vi "Moxom.vi"() -> ()   [LabVIEW 2011]
doc: "This the Rose-Hulman Robotics Tream IGVC compatition Code\nexample demonstrates the control of an autonomous robot through multiple asynchronous processes, modeled by VIs, that communicate with each other using shared variables. This example also shows an obstacle avoidance algorithm that the simulated robot uses as it navigates. The application includes the following processes:\n\n1. LIDAR Loop (\"Sense\")--Uses LabVIEW dataflow programming to generate simulated sensor data based on the position of the robot and any obstacles in the environment.\n\n2. Operator Loop (\"Think\")--Uses a state machine to control the movement of the robot according to commands from the user. When the robot follows a path without joystick or keyboard control, this process controls the attitude of the autonomous robot using a Vector Field Histogram (VFH) algorithm to avoid obstacles.\n\n3. Motor Loop (\"Act\")--Uses a Control and Simulation Loop, from the Control Design and Simulation Module, to create a model of the robot, simulate its dynamic behavior, and show the control loops and attitude observers."
uses:
  <vilib>/robotics/Controls/Compass Indicator/Compass Indicator.xctl
  <vilib>/Platform/TimedLoop/XDataNode/timing_clust.ctl
  <vilib>/Platform/TimedLoop/XDataNode/nitl_modes.ctl
  <vilib>/Platform/TimedLoop/XDataNode/wakeup.ctl
  <vilib>/Platform/TimedLoop/XDataNode/XDataNode.xnode
  <vilib>/Platform/TimedLoop/XDataNode/XDNodeRunTimeDep.lvlib
panel:
  out "Error":bool
  out "OK":bool
  in  "HUD 2":enum32{"GPS", "LIDAR", "IMU", "Occupancy Grid"}(tab)
  out "Health":u8(slide) scale=0.0..12.0
  out "XY Graph 2":cluster{dbl[], dbl[]}(graph)
  out "Data Aquired 2":picture
  out "Digree 2":dbl=16.3201904296875 caption="Digree"
  out "Compass Indicator 2":dbl(xcontrol)=16.3201904296875
  out "Occupancy Grid":dbl[][](graph)
  in  "Telemetry":T1(tab)
  out "Voltage":cluster{sgl, sgl, sgl}(knob)={13.4, 12.0, 47.48} caption="Main Battery Voltage\nInternal Voltage\nDSUB Voltage" scale=8.0..15.0
  out "Current":cluster{sgl, sgl, sgl, sgl}(knob)={0.0, 0.0, -2.0, -2.0} caption="Ch1 Motor Curret\nCh2 Motor Curret\nCh1 Battery Curret \nCh2 Battery Curret" scale=0.0..15.0
  out "IC Temp (C)":i32(slide)=22 scale=0.0..150.0
  out "Ch1 Temp (C)":i32(slide)=22 scale=0.0..150.0
  out "Ch2 Temp (C)":i32(slide)=23 scale=0.0..150.0
  out "Ch1 Encoder Speed\nCh2 Encoder Speed":cluster{i32, i32}(knob) scale=-300.0..300.0
  out "Image Out":T2(plugin-control)
  in  "Search For VISA":bool
  in  "Max RPM/Effort":i32(slide) scale=0.0..1000.0
  in  "HUD":T3(tab)=enum."Info"
  in  "Analog Stick":cluster{dbl, dbl}[](graph)
  in  "Clear Breadcrumbs":bool
  in  "Max Points":dbl=3000.0 format="%0.2f"
  out "XY Graph":cluster{dbl[], dbl[]}[](graph)
  out "Longitude Point":dbl format="%#_12g"
  out "Latitude Point":dbl format="%#_12g"
  out "Data Aquired":picture
  in  "Max Distance":dbl=3000.0 format="%0.2f"
  out "Digree":dbl=16.3201904296875
  out "Compass Indicator":dbl(xcontrol)=16.3201904296875
  out "Curretn POI":string
  in  "Curent Index":i32
  in  "Waypoint Table":string[][](table)=[["1.000000", "39.400000", "-87.200000"], ["2.000000", "39.600000", "-87.300000"], ["2.000000", "39.200000", "-87.400000"]]
  in  "Show GPS Diagram":bool
  in  "Show LL Diagram":bool
  in  "Show OL Diagram":bool
  in  "Show MCL Diagram":bool
  in  "VFH Visualization":bool
  in  "About":bool
  in  "Stop":bool
  in  "Error Display":T4(tab)
  out "Cammera Status":bool
  out "Cammera Status 2":bool
  out "IMU Status":bool
  in  "IMU VISA":refnum<visa-resource-name>="COM7"
  out "Motor Status":bool
  in  "Motor VISA":refnum<visa-resource-name>="COM21"
  out "LIDAR Status":bool
  in  "LIDAR VISA":refnum<visa-resource-name>="COM20"
  out "GPS Status":bool
  in  "GPS VISA":refnum<visa-resource-name>="COM22"
  in  "GPS Error":errorcluster
  in  "LIDAR Error":errorcluster
  in  "Motor Error":errorcluster
  in  "IMU Error":errorcluster
  in  "Camera Error":errorcluster
  in  "Robot Mode:":T5(ring)
  out "End Loop":bool=TRUE
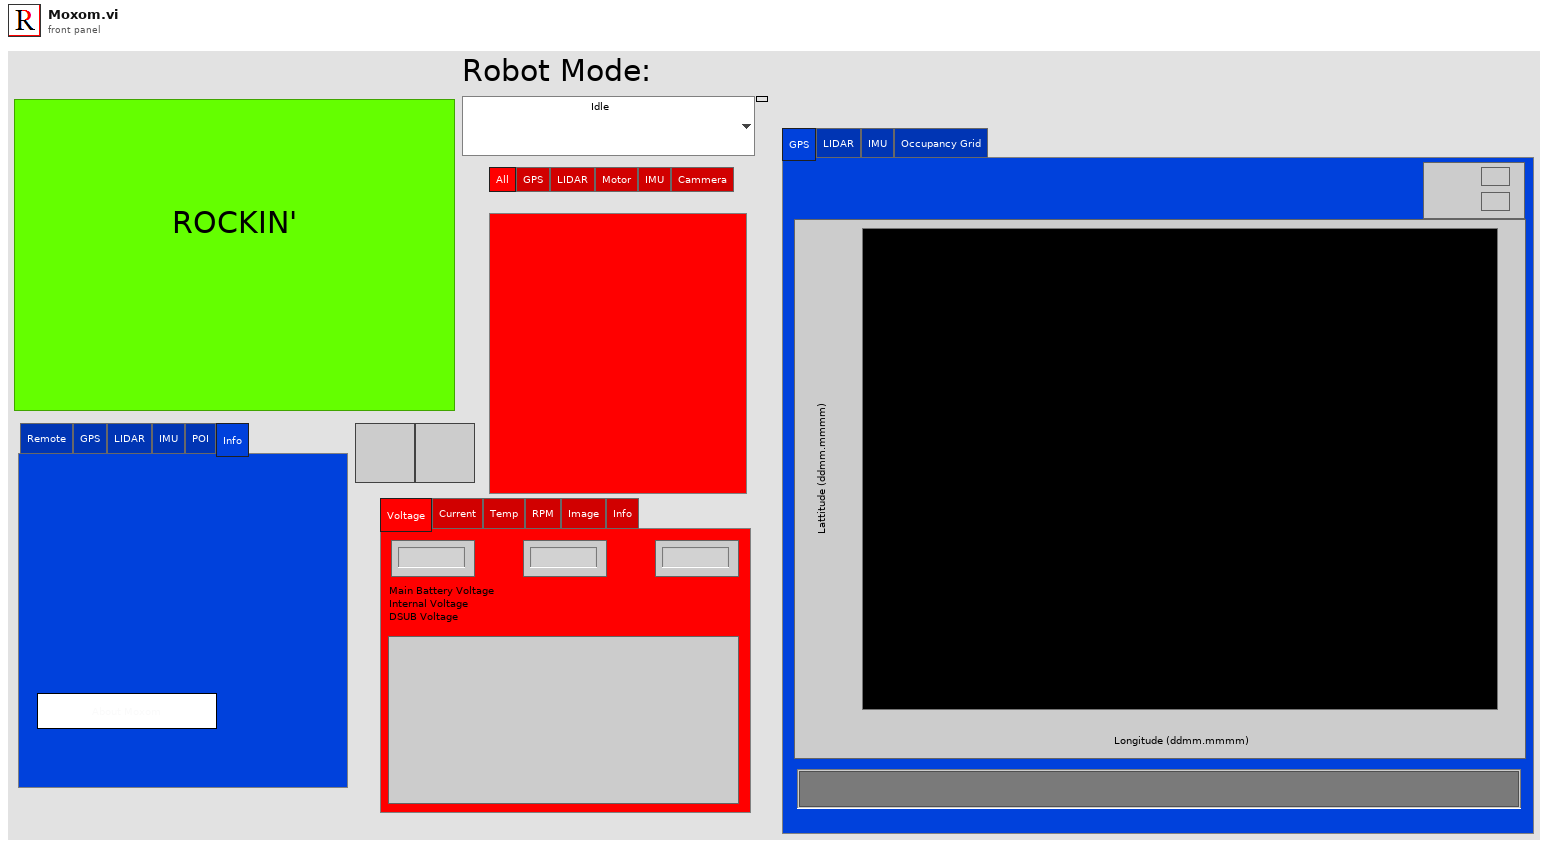
[diagram p1: front panel]
types:
  T1 = enum32{"Voltage", "Current", "Temp", "RPM", "Image", "Info"}
  T2 = typedef "IMAQ Image.ctl" = refnum<image>
  T3 = enum32{"Remote", "GPS", "LIDAR", "IMU", "POI", "Info"}
  T4 = enum32{"All", "GPS", "LIDAR", "Motor", "IMU", "Cammera"}
  T5 = enum16{"Idle", "Wiimote", "Joypad", "IGVC", "Avoide Objects", "Avoide Lines", "Path Planning", "Heading", "Waypoint"}
  T6 = cluster{"Latitude":dbl, "Longitude":dbl, "Altitude":dbl, "Velocity, Correction & SET":cluster{"Velocity North":dbl, "Velocity East":dbl, "Velocity Up":dbl, "Ellipsoidal Height":dbl, "GDOP":sgl, "PDOP":sgl, "HDOP":sgl, "VDOP":sgl, "TDOP":sgl, "Horizontal Figure of Merit":u8, "Time Figure of Merit":u8, "Max dGPS Age":sgl, "Extended Navigation Mode":u8, "Antenna Height Adjustment ":dbl, "SET North":i32, "SET East":i32, "SET Up":i32}, "Time":cluster{"GPS Week":u16, "GPS Time of Week":sgl}, "Satellites Used":i32[]}
  T7 = typedef "XDNodeRunTimeDep.lvlib/timing_clust.ctl" = cluster{"Expected End [f-1]":u64, "Actual End [f-1]":u64, "Finished Late? [f-1]":bool, "Expected End [i-1]":u64, "Actual End [i-1]":u64, "Finished Late? [i-1]":bool, "Expected Start [i]":u64, "Actual Start [i]":u64, "Expected Start [f]":u64, "Actual Start [f]":u64, "Source Name":string, "Structure Name":string, "Period":i64, "Deadline":i64, "Offset":i64, "Start":i64, "Priority":i32, "Timeout":i32, "Mode":T8, "Wakeup Reason":T9, "Error":errorcluster, "Source Type":string, "Secondary Source Type":string, "Global End Time":u64, "Global Start Time":u64, "Frame Duration":u64, "Iteration Duration":u64, "Assigned CPU":i32, "I/O Scan Engine Mode":u32}
  T8 = typedef "XDNodeRunTimeDep.lvlib/nitl_modes.ctl" = enum32{"No Change", "Process missed periods, maintain original phase", "Discard missed periods, maintain original phase", "Process missed periods, ignore original phase", "Discard missed periods, ignore original phase"}
  T9 = typedef "XDNodeRunTimeDep.lvlib/wakeup.ctl" = enum32{"Normal", "Aborted", "Asynchronous wakeup", "Timing source error", "Timed loop error", "Timeout"}
  T10 = cluster{"Position":cluster{"Roll":dbl, "Pitch":dbl, "Yaw":dbl}, "Orientation Matrix":dbl[][], "Magnetic Field":cluster{"Z-Axis Magnetic Field":dbl, "Y-Axis Magnetic Field":dbl, "X-Axis Magnetic Field":dbl}, "Acceleration":cluster{"Z-Axis Acceleration":dbl, "Y-Axis Acceleration":dbl, "X-Axis Acceleration":dbl}, "Angular Rate":cluster{"X-Axis Angular Rate":dbl, "Y-Axis Angular Rate":dbl, "Z-Axis Angular Rate":dbl}, "Quaternion":dbl[]}
  T11 = cluster{"Azimuth":dbl, "FocusPointAltitude":dbl, "altMode":i32, "FocusPointLatitude":dbl, "FocusPointLongitude":dbl, "Range":dbl, "Tilt":dbl}
  T12 = cluster{"Voltage":cluster{sgl, sgl, sgl}, "Encoder Speed":cluster{i32, i32}, "Temps":cluster{"IC Temp (C)":i32, "Ch1 Temp (C)":i32, "Ch2 Temp (C)":i32}, "Current":cluster{dbl, dbl, dbl, dbl}}
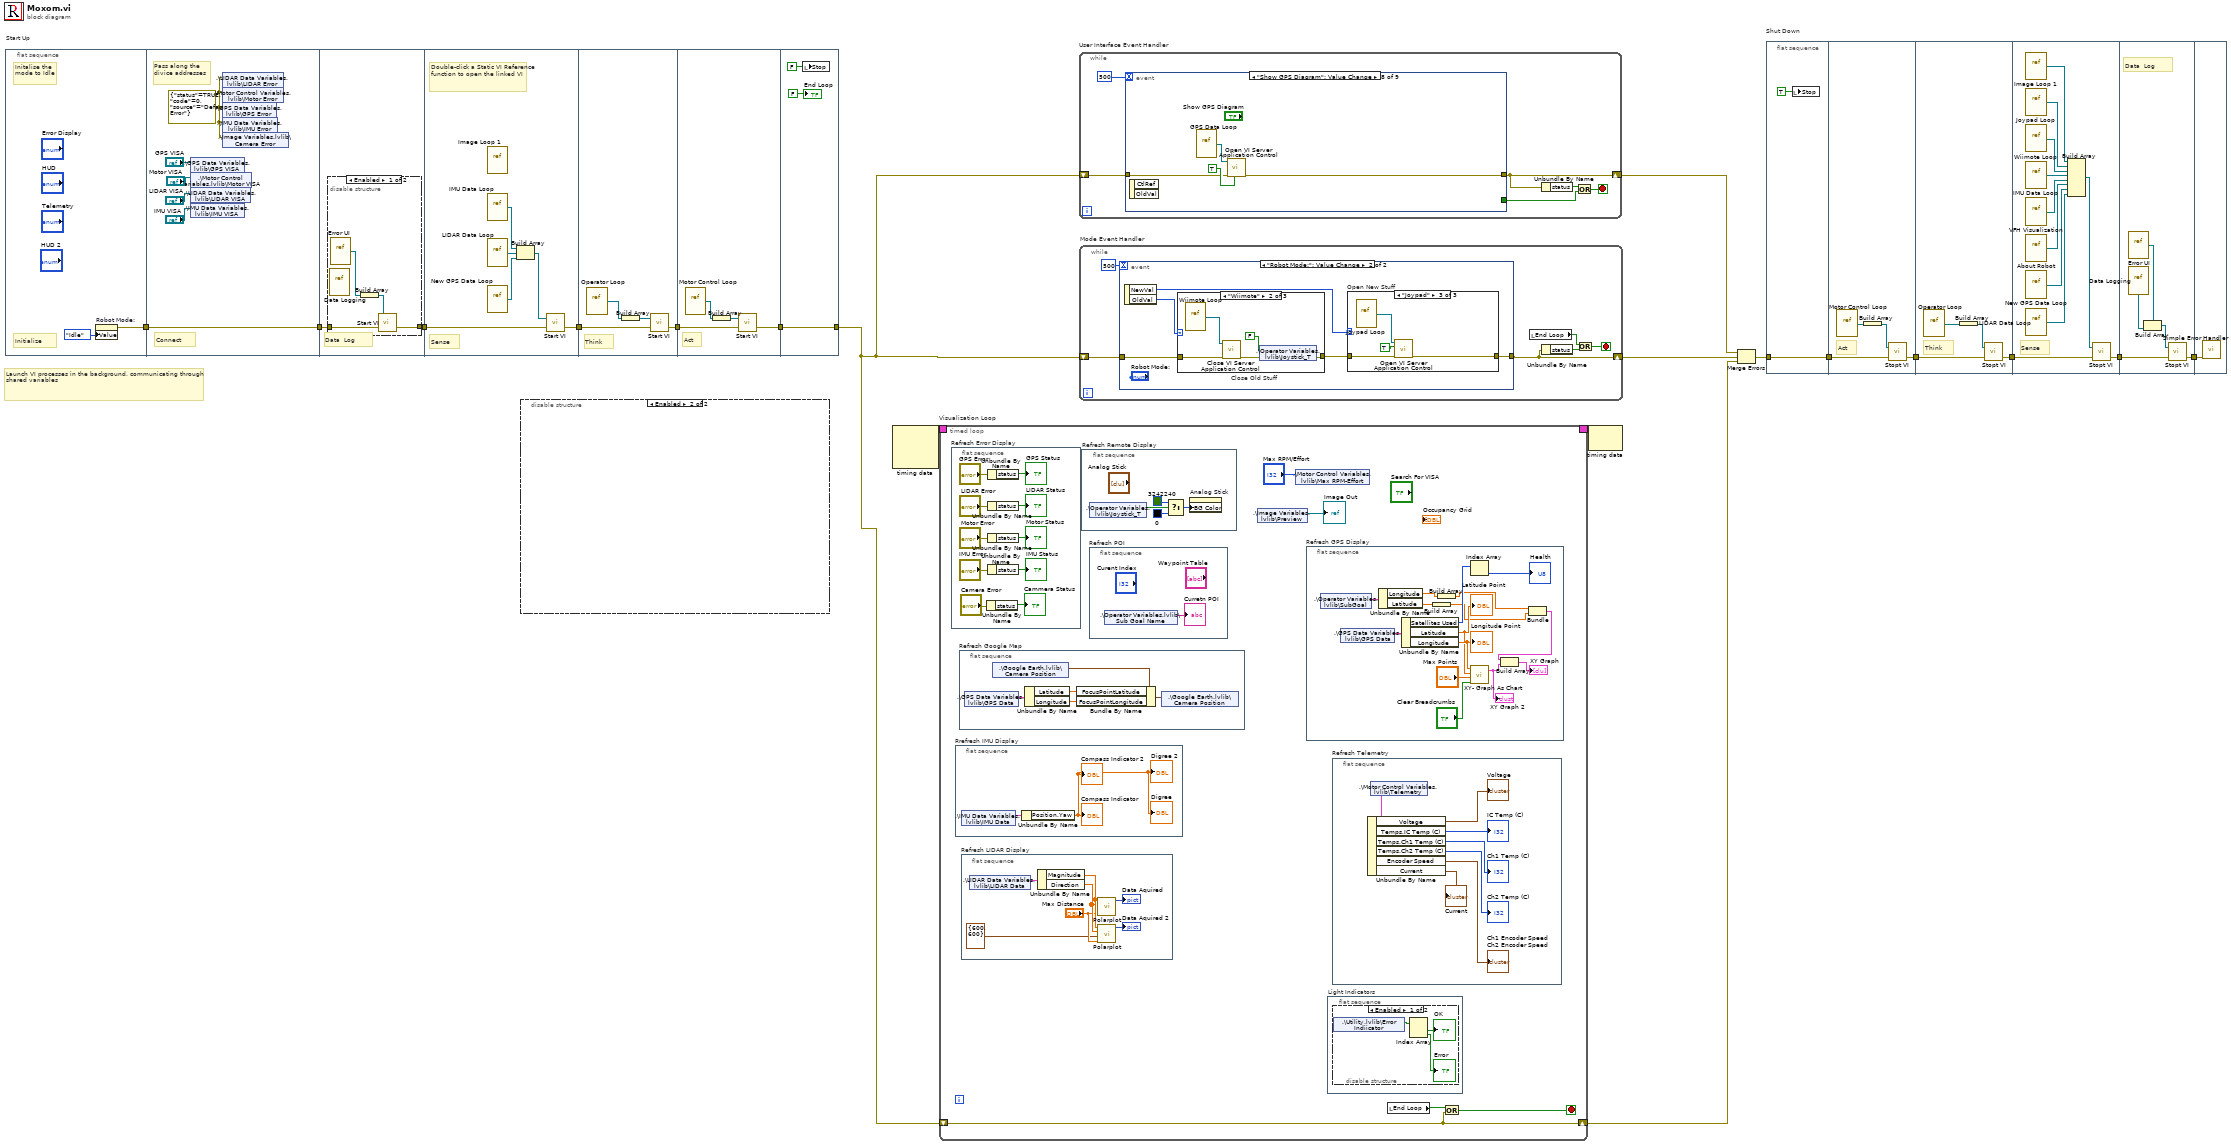
[diagram p0: block diagram]
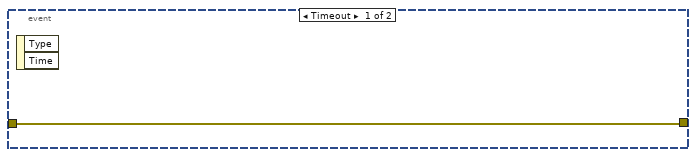
[diagram p2: hidden frame]
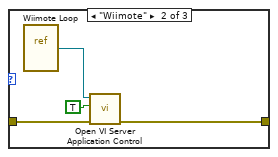
[diagram p4: hidden frame]
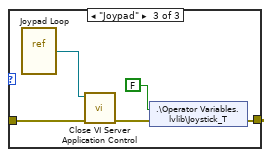
[diagram p6: hidden frame]
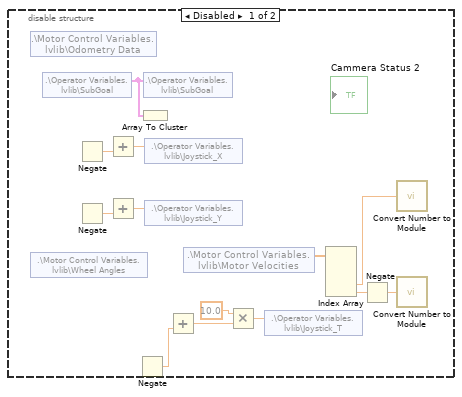
[diagram p7: hidden frame]
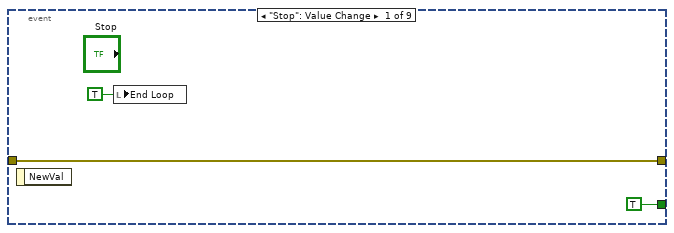
[diagram p9: hidden frame]
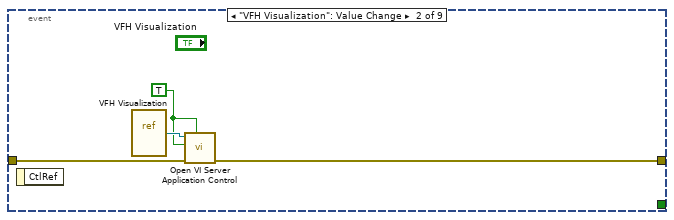
[diagram p10: hidden frame]
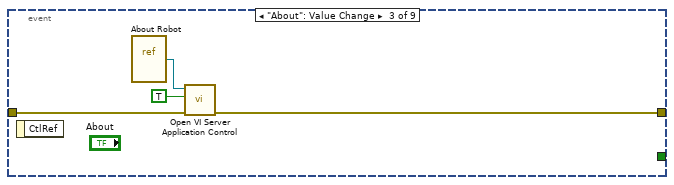
[diagram p11: hidden frame]
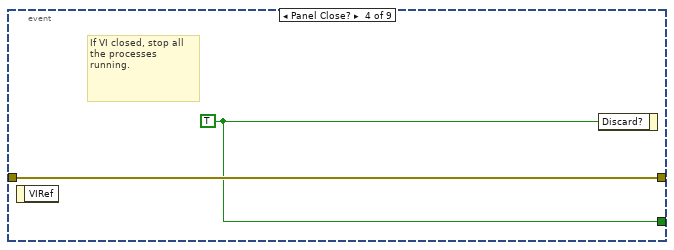
[diagram p12: hidden frame]
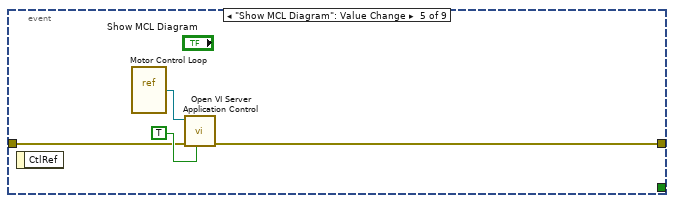
[diagram p13: hidden frame]
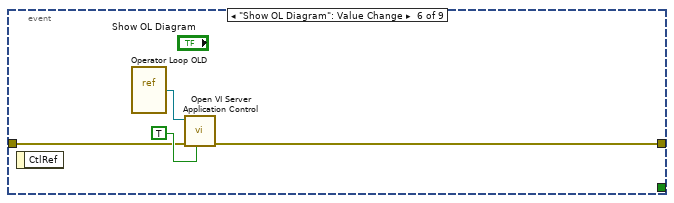
[diagram p14: hidden frame]
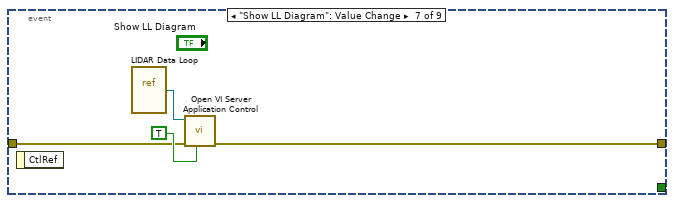
[diagram p15: hidden frame]
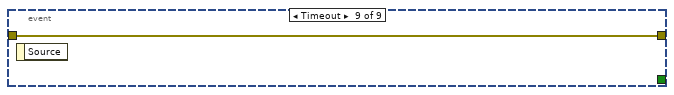
[diagram p16: hidden frame]
diagram:
  # "Launch VI processes in the background, communicating through shared variables"
  n1 = flat-sequence "Start Up" {
    tunnel: [w20] -> w13
    tunnel: [w23] -> w5
    tunnel: w13 -> [w23]
    tunnel: w5 -> [w28]
    tunnel: [w27] -> w1
    tunnel: [w37] -> w12
    tunnel: w1 -> [w38]
    tunnel: w12 -> [w43]
    tunnel: [w42] -> w10
    tunnel: [w46] -> w11
    tunnel: w10 -> [w47]
    tunnel: [w50] -> w6
    tunnel: w11 -> [w50]
    frame #0 {
      # "Initialize"
      # "Initalise the mode to Idle"
      n2 = property on="Robot Mode:" class="Enum (strict)"("Value"=T5."Idle" ("Robot Mode:")) -> (error out=w20:errorcluster)  [unwired: 2 in, 1 out]
    }
    frame #1 {
      w21 = errorcluster {"status"=TRUE, "code"=0, "source"="Default Error"} ("error out")
      # "Connect"
      # "Pass along the divice addresses"
      n3 = shared-variable ".\\GPS Data Variables.lvlib\\GPS VISA"("GPS VISA") -> ()  [unwired: 1 in, 1 out]
      n4 = shared-variable ".\\LIDAR Data Variables.lvlib\\LIDAR VISA"("LIDAR VISA") -> ()  [unwired: 1 in, 1 out]
      n5 = shared-variable ".\\IMU Data Variables.lvlib\\IMU VISA"("IMU VISA") -> ()  [unwired: 1 in, 1 out]
      n6 = shared-variable ".\\Motor Control Variables.lvlib\\Motor VISA"("Motor VISA") -> ()  [unwired: 1 in, 1 out]
      n7 = shared-variable ".\\LIDAR Data Variables.lvlib\\LIDAR Error"(w21) -> ()  [unwired: 1 in, 1 out]
      n8 = shared-variable ".\\Motor Control Variables.lvlib\\Motor Error"(w21) -> ()  [unwired: 1 in, 1 out]
      n9 = shared-variable ".\\GPS Data Variables.lvlib\\GPS Error"(w21) -> ()  [unwired: 1 in, 1 out]
      n10 = shared-variable ".\\IMU Data Variables.lvlib\\IMU Error"(w21) -> ()  [unwired: 1 in, 1 out]
      n11 = shared-variable ".\\Image Variables.lvlib\\Camera Error"(w21) -> ()  [unwired: 1 in, 1 out]
    }
    frame #2 {
      # "Data  Log"
      n12 = disable-structure shown="Enabled" {
        disable-tunnel: w28 -> [w31 w33]
        disable-tunnel: [w30 w33] -> w27
        frame Enabled {
          n13 = vi-ref "Data Logging.vi"() -> ()  [unwired: 1 out]
          n14 = vi-ref "Error UI.vi"() -> (w29:refnum<vi>)
          n15 = Build Array(w29) -> (w32:refnum<vi>[])
          n16 = call "Start VI.vi"("error in"=w31, "VI refnum"=w32) -> ("error out"=w30:errorcluster)  [unwired: 1 in]
        }
        frame Disabled {
        }
      }
    }
    frame #3 {
      # "Double-click a Static VI Reference function to open the linked VI"
      # "Sense"
      n17 = vi-ref "Image Loop 1.vi"() -> ()  [unwired: 1 out]
      n18 = vi-ref "IMU Data Loop.vi"() -> (w35:refnum<vi>)
      n19 = vi-ref "LIDAR Data Loop.vi"() -> (w36:refnum<vi>)
      n20 = vi-ref "New GPS Data Loop.vi"() -> (w34:refnum<vi>)
      n21 = Build Array(w35, w36, w34) -> (w39:refnum<vi>[])
      n22 = call "Start VI.vi"("error in"=w38, "VI refnum"=w39) -> ("error out"=w37:errorcluster)  [unwired: 1 in]
    }
    frame #4 {
      # "Think"
      n23 = vi-ref "Operator Loop.vi"() -> (w41:refnum<vi>)
      n24 = Build Array(w41) -> (w40:refnum<vi>[])
      n25 = call "Start VI.vi"("error in"=w43, "VI refnum"=w40) -> ("error out"=w42:errorcluster)  [unwired: 1 in]
    }
    frame #5 {
      # "Act"
      n26 = vi-ref "Motor Control Loop.vi"() -> (w45:refnum<vi>)
      n27 = Build Array(w45) -> (w44:refnum<vi>[])
      n28 = call "Start VI.vi"("error in"=w47, "VI refnum"=w44) -> ("error out"=w46:errorcluster)  [unwired: 1 in]
    }
    frame #6 {
      n29 = local write "Stop"(FALSE ("Halt TL")) -> ()
      "End Loop" <- FALSE ("Halt TL")
    }
  }
  n30 = disable-structure shown="Enabled" {
    frame Disabled {
      n31 = shared-variable ".\\Motor Control Variables.lvlib\\Odometry Data"() -> ()  [unwired: 1 in, 2 out]
      n32 = shared-variable ".\\Motor Control Variables.lvlib\\Wheel Angles"() -> ()  [unwired: 1 in, 2 out]
      n33 = shared-variable ".\\Operator Variables.lvlib\\SubGoal"() -> (w51:T6)  [unwired: 1 in, 1 out]
      n34 = Negate() -> (-x=w55:dbl)  [unwired: 1 in]
      n35 = Negate() -> (-x=w56:dbl)  [unwired: 1 in]
      n36 = Add(y=w55) -> (x+y=w65:dbl)  [unwired: 1 in]
      n37 = Add(y=w56) -> (x+y=w64:dbl)  [unwired: 1 in]
      n38 = Negate() -> (-x=w54:dbl)  [unwired: 1 in]
      n39 = Array To Cluster(array=w51) -> ()  [unwired: 1 out]
      n40 = shared-variable ".\\Operator Variables.lvlib\\SubGoal"(w51) -> ()  [unwired: 1 in, 1 out]
      n41 = shared-variable ".\\Operator Variables.lvlib\\Joystick_X"(w65) -> ()  [unwired: 1 in, 1 out]
      n42 = shared-variable ".\\Operator Variables.lvlib\\Joystick_Y"(w64) -> ()  [unwired: 1 in, 1 out]
      n43 = Add(y=w54) -> (x+y=w53:dbl)  [unwired: 1 in]
      n44 = shared-variable ".\\Motor Control Variables.lvlib\\Motor Velocities"() -> (w62:dbl[])  [unwired: 1 in, 1 out]
      n45 = Multiply(x=10.0, y=w53) -> (x*y=w63:dbl)
      n46 = shared-variable ".\\Operator Variables.lvlib\\Joystick_T"(w63) -> ()  [unwired: 1 in, 1 out]
      n47 = Index Array(array=w62) -> (element #3=w59:dbl, element #4=w58:dbl)  [unwired: 4 in, 2 out]
      n48 = Negate(x=w58) -> (-x=w57:dbl)
      n49 = call "Convert Number to Module.vi"("input"=w59) -> ("Positive Module"=w60:dbl)  [unwired: 6 in, 1 out]
      n50 = call "Convert Number to Module.vi"("input"=w57) -> ("Positive Module"=w61:dbl)  [unwired: 6 in, 1 out]
    }
    frame Enabled {
    }
  }
  n51 = node-c288() -> (w18:T7)  [unwired: 3 in]
  n52 = timed-loop "Visualization Loop" {
    timing: w18 -> [_]
    timing-out: [_] -> w17
    shift-right: [w66] -> w2
    shift-left: w6 -> [w66]
    stop <- w70 stop-if-true
    n53 = flat-sequence "Refresh Error Display" {
      frame #0 {
        n54 = Unbundle By Name("Camera Error") -> ("status"=→"Cammera Status":bool)
        n55 = Unbundle By Name("GPS Error") -> ("status"=→"GPS Status":bool)
        n56 = Unbundle By Name("LIDAR Error") -> ("status"=→"LIDAR Status":bool)
        n57 = Unbundle By Name("Motor Error") -> ("status"=→"Motor Status":bool)
        n58 = Unbundle By Name("IMU Error") -> ("status"=→"IMU Status":bool)
      }
    }
    n59 = flat-sequence "Rrefresh IMU Display" {
      frame #0 {
        n60 = shared-variable ".\\IMU Data Variables.lvlib\\IMU Data"() -> (w98:T10)  [unwired: 1 in, 1 out]
        n61 = Unbundle By Name(w98) -> ("Position.Yaw"=→"Compass Indicator" →"Digree" →"Compass Indicator 2" →"Digree 2":dbl)
      }
    }
    n62 = flat-sequence "Refresh Google Map" {
      frame #0 {
        n63 = shared-variable ".\\GPS Data Variables.lvlib\\GPS Data"() -> (w109:T6)  [unwired: 1 in, 1 out]
        n64 = shared-variable ".\\Google Earth.lvlib\\Camera Position"() -> (w110:T11)  [unwired: 1 in, 1 out]
        n65 = Unbundle By Name(w109) -> ("Latitude"=w106:dbl, "Longitude"=w108:dbl)
        n66 = Bundle By Name(cluster=w110, "FocusPointLatitude"=w106, "FocusPointLongitude"=w108) -> (w107:T11)
        n67 = shared-variable ".\\Google Earth.lvlib\\Camera Position"(w107) -> ()  [unwired: 1 in, 1 out]
      }
    }
    n68 = flat-sequence "Refresh LIDAR Display" {
      frame #0 {
        n69 = shared-variable ".\\LIDAR Data Variables.lvlib\\LIDAR Data"() -> (w80:cluster{"Magnitude":dbl[], "Direction":dbl[]})  [unwired: 1 in, 1 out]
        n70 = Unbundle By Name(w80) -> ("Magnitude"=w77:dbl[], "Direction"=w76:dbl[])
        n71 = call "Polarplot.vi"("maximum"="Max Distance", "Direction"=w76, "Magnitude"=w77) -> ("Data Aquired"=→"Data Aquired":picture)  [unwired: 8 in]
        n72 = call "Polarplot.vi"("maximum"="Max Distance", "dimensions (w,h)"=cluster{"width":i16, "height":i16} {"width"=600, "height"=600}, "Direction"=w76, "Magnitude"=w77) -> ("Data Aquired"=→"Data Aquired 2":picture)  [unwired: 7 in]
      }
    }
    n73 = flat-sequence "Refresh Remote Display" {
      frame #0 {
        n74 = shared-variable ".\\Operator Variables.lvlib\\Joystick_T"() -> (w112:bool)  [unwired: 1 in, 1 out]
        n75 = Select(t=u32 3242240, s=w112, f=u32 0) -> (s? t:f=w111:u32)
        n76 = property on="Analog Stick" class="XYGraph (strict)"("BG Color"=w111) -> ()  [unwired: 2 in, 2 out]
      }
    }
    n77 = flat-sequence "Refresh POI" {
      frame #0 {
        n78 = shared-variable ".\\Operator Variables.lvlib\\Sub Goal Name"() -> (→"Curretn POI":string)  [unwired: 1 in, 1 out]
      }
    }
    n79 = shared-variable ".\\Image Variables.lvlib\\Preview"() -> (→"Image Out":refnum<image>)  [unwired: 1 in, 1 out]
    n80 = shared-variable ".\\Motor Control Variables.lvlib\\Max RPM-Effort"("Max RPM/Effort") -> ()  [unwired: 1 in, 1 out]
    n81 = flat-sequence "Refresh GPS Display" {
      frame #0 {
        n82 = shared-variable ".\\Operator Variables.lvlib\\SubGoal"() -> (w91:T6)  [unwired: 1 in, 1 out]
        n83 = shared-variable ".\\GPS Data Variables.lvlib\\GPS Data"() -> (w95:T6)  [unwired: 1 in, 1 out]
        n84 = Unbundle By Name(w91) -> ("Longitude"=w86:dbl, "Latitude"=w85:dbl)
        n85 = Unbundle By Name(w95) -> ("Satellites Used"=w92:i32[], "Latitude"=w89:dbl, "Longitude"=w90:dbl)
        "Latitude Point" <- w89
        "Longitude Point" <- w90
        n86 = Build Array(w85) -> (w83:dbl[])
        n87 = Build Array(w86) -> (w84:dbl[])
        n88 = Index Array(array=w92) -> (element=→"Health":i32)  [unwired: 1 in]
        n89 = call "XY- Graph As Chart.vi"("Clear Graph (F)"="Clear Breadcrumbs", "Maxi Points (10,000)"="Max Points", "Y-Value"=w89, "X- Value"=w90) -> ("XY Graph"=w88:cluster{dbl[], dbl[]})  [unwired: 1 out]
        "XY Graph 2" <- w88
        n90 = Bundle(w84, w83) -> (w82:cluster{dbl[], dbl[]})  [unwired: 1 out]
        n91 = Build Array(w82, w88) -> (→"XY Graph":cluster{dbl[], dbl[]}[])
      }
    }
    n92 = flat-sequence "Light Indicators" {
      frame #0 {
        n93 = disable-structure shown="Enabled" {
          frame Enabled {
            n94 = shared-variable ".\\Utility.lvlib\\Error Indiicator"() -> (w73:bool[])  [unwired: 1 in, 1 out]
            n95 = Index Array(array=w73) -> (element #1=→"OK":bool, element #2=→"Error":bool)  [unwired: 2 in]
          }
          frame Disabled {
          }
        }
      }
    }
    n96 = flat-sequence "Refresh Telemetry" {
      frame #0 {
        n97 = shared-variable ".\\Motor Control Variables.lvlib\\Telemetry"() -> (w105:T12)  [unwired: 1 in, 1 out]
        n98 = Unbundle By Name(w105) -> ("Voltage"=→"Voltage":cluster{sgl, sgl, sgl}, "Temps.IC Temp (C)"=→"IC Temp (C)":i32, "Temps.Ch1 Temp (C)"=→"Ch1 Temp (C)":i32, "Temps.Ch2 Temp (C)"=→"Ch2 Temp (C)":i32, "Encoder Speed"=→"Ch1 Encoder Speed\nCh2 Encoder Speed":cluster{i32, i32}, "Current"=→"Current":cluster{dbl, dbl, dbl, dbl})
      }
    }
    n99 = local read "End Loop"() -> (w67:bool)
    n100 = Or(x=w67, y=w66) -> (x .or. y?=w70:bool)
  }
  n101 = while "User Interface Event Handler" {
    shift-right: [w129] -> w16
    shift-left: w6 -> [w132]
    stop <- w131 stop-if-true
    n102 = event shown="[7] \"Show GPS Diagram\": Value Change" {
      selector: _ -> [_ _ _ _ _ _ _ _ _]
      dyn-events: _ -> [_ _ _ _ _ _ _ _ _]
      timeout: 500 -> [_ _ _ _ _ _ _ _ _]
      tunnel: [TRUE _ _ w144 _ _ _ _ _] -> w127
      tunnel: w132 -> [w135 w137 w142 w145 w147 w151 w155 w158 w162]
      tunnel: [w135 w136 w141 w145 w146 w150 w154 w159 w162] -> w129
      event "Stop": Value Change {
        n103 = event-data() -> ()  [unwired: 2 out]
        n104 = local write "End Loop"(TRUE ("End Loop")) -> ()
      }
      event "VFH Visualization": Value Change {
        w138 = TRUE ("Launch Map")
        n105 = event-data() -> ()  [unwired: 2 out]
        n106 = vi-ref "VFH Visualization.vi"() -> (w139:refnum<vi>)
        n107 = call "Open VI Server Application Control.vi"("open front panel (F)"=w138, "error in (no error)"=w137, "run VI (F)"=w138, "VI refnum"=w139) -> ("error out"=w136:errorcluster)  [unwired: 7 in]
      }
      event "About": Value Change {
        n108 = event-data() -> ()  [unwired: 2 out]
        n109 = vi-ref "About Robot.vi"() -> (w143:refnum<vi>)
        n110 = call "Open VI Server Application Control.vi"("error in (no error)"=w142, "run VI (F)"=TRUE ("Launch Map"), "VI refnum"=w143) -> ("error out"=w141:errorcluster)  [unwired: 8 in]
      }
      event Panel Close? {
        w144 = TRUE ("Discard?")
        # "If VI closed, stop all the processes running."
        n111 = event-data() -> ()  [unwired: 2 out]
        n112 = event-data("Discard?"=w144) -> ()  [unwired: 1 in, 1 out]
      }
      event "Show MCL Diagram": Value Change {
        n113 = event-data() -> ()  [unwired: 2 out]
        n114 = vi-ref "Motor Control Loop.vi"() -> (w149:refnum<vi>)
        n115 = call "Open VI Server Application Control.vi"("open block diagram (F)"=TRUE ("Open Front Panel"), "error in (no error)"=w147, "VI refnum"=w149) -> ("error out"=w146:errorcluster)  [unwired: 8 in]
      }
      event "Show OL Diagram": Value Change {
        n116 = event-data() -> ()  [unwired: 2 out]
        n117 = vi-ref "Operator Loop OLD.vi"() -> (w152:refnum<vi>)
        n118 = call "Open VI Server Application Control.vi"("open block diagram (F)"=TRUE ("Open Front Panel"), "error in (no error)"=w151, "VI refnum"=w152) -> ("error out"=w150:errorcluster)  [unwired: 8 in]
      }
      event "Show LL Diagram": Value Change {
        n119 = event-data() -> ()  [unwired: 2 out]
        n120 = vi-ref "LIDAR Data Loop.vi"() -> (w156:refnum<vi>)
        n121 = call "Open VI Server Application Control.vi"("open block diagram (F)"=TRUE ("Open Front Panel"), "error in (no error)"=w155, "VI refnum"=w156) -> ("error out"=w154:errorcluster)  [unwired: 8 in]
      }
      event "Show GPS Diagram": Value Change {
        n122 = event-data() -> ()  [unwired: 3 out]
        n123 = vi-ref "GPS Data Loop.vi"() -> (w160:refnum<vi>)
        n124 = call "Open VI Server Application Control.vi"("open block diagram (F)"=TRUE ("Open Front Panel"), "error in (no error)"=w158, "VI refnum"=w160) -> ("error out"=w159:errorcluster)  [unwired: 8 in]
      }
      event Timeout {
        n125 = event-data() -> ()  [unwired: 2 out]
      }
    }
    n126 = Unbundle By Name(w129) -> ("status"=w128:bool)
    n127 = Or(x=w128, y=w127) -> (x .or. y?=w131:bool)
  }
  n128 = while "Mode Event Handler" {
    shift-right: [w165] -> w7
    shift-left: w6 -> [w166]
    stop <- w167 stop-if-true
    n129 = event shown="[1] \"Robot Mode:\": Value Change" {
      selector: _ -> [_ _]
      dyn-events: _ -> [_ _]
      timeout: 500 -> [_ _]
      tunnel: [w169 w172] -> w165
      tunnel: w166 -> [w169 w174]
      event Timeout {
        n130 = event-data() -> ()  [unwired: 1 in, 2 out]
      }
      event "Robot Mode:": Value Change {
        n131 = event-data() -> ("NewVal"=w171:T5, "OldVal"=w170:T5)  [unwired: 1 in]
        n132 = case "Close Old Stuff" shown="\"Wiimote\"" w170 {
          tunnel: w174 -> [w184 w189 w194]
          tunnel: [w184 w185 w190] -> w173
          frame "Idle", Default {
          }
          frame "Wiimote" {
            n133 = vi-ref "Wiimote Loop.vi"() -> (w188:refnum<vi>)
            n134 = call "Close VI Server Application Control.vi"("error in (no error)"=w189, "VI refnum"=w188) -> ("error out"=w186:errorcluster)  [unwired: 9 in]
            n135 = shared-variable ".\\Operator Variables.lvlib\\Joystick_T"(FALSE ("Joystick_T"), error in=w186) -> (error out=w185:errorcluster)
          }
          frame "Joypad" {
            n136 = vi-ref "Joypad Loop.vi"() -> (w193:refnum<vi>)
            n137 = call "Close VI Server Application Control.vi"("error in (no error)"=w194, "VI refnum"=w193) -> ("error out"=w191:errorcluster)  [unwired: 9 in]
            n138 = shared-variable ".\\Operator Variables.lvlib\\Joystick_T"(FALSE ("Joystick_T"), error in=w191) -> (error out=w190:errorcluster)
          }
        }
        n139 = case "Open New Stuff" shown="\"Joypad\"" w171 {
          tunnel: w173 -> [w175 w179 w183]
          tunnel: [w175 w177 w181] -> w172
          frame "Idle", Default {
          }
          frame "Wiimote" {
            n140 = vi-ref "Wiimote Loop.vi"() -> (w176:refnum<vi>)
            n141 = call "Open VI Server Application Control.vi"("error in (no error)"=w179, "run VI (F)"=TRUE, "VI refnum"=w176) -> ("error out"=w177:errorcluster)  [unwired: 8 in]
          }
          frame "Joypad" {
            n142 = vi-ref "Joypad Loop.vi"() -> (w180:refnum<vi>)
            n143 = call "Open VI Server Application Control.vi"("error in (no error)"=w183, "run VI (F)"=TRUE, "VI refnum"=w180) -> ("error out"=w181:errorcluster)  [unwired: 8 in]
          }
        }
      }
    }
    n144 = local read "End Loop"() -> (w164:bool)
    n145 = Unbundle By Name(w165) -> ("status"=w168:bool)
    n146 = Or(x=w164, y=w168) -> (x .or. y?=w167:bool)
  }
  n147 = node-c288(w17) -> ()  [unwired: 1 out]
  n148 = Merge Errors(w16, w7, w2) -> (w14:errorcluster)
  n149 = flat-sequence "Shut Down" {
    tunnel: w14 -> [w195]
    tunnel: [w195] -> w15
    tunnel: w15 -> [w200]
    tunnel: [w199] -> w9
    tunnel: w9 -> [w204]
    tunnel: [w203] -> w8
    tunnel: w8 -> [w215]
    tunnel: [w214] -> w4
    tunnel: w4 -> [w217]
    tunnel: [w220] -> w3
    tunnel: w3 -> [w221]
    frame #0 {
      n150 = local write "Stop"(TRUE ("Halt TL")) -> ()
    }
    frame #1 {
      # "Act"
      n151 = vi-ref "Motor Control Loop.vi"() -> (w198:refnum<vi>)
      n152 = Build Array(w198) -> (w197:refnum<vi>[])
      n153 = call "Stopt VI.vi"("error in"=w200, "VI refnum"=w197) -> ("error out"=w199:errorcluster)  [unwired: 1 in]
    }
    frame #2 {
      # "Think"
      n154 = vi-ref "Operator Loop.vi"() -> (w201:refnum<vi>)
      n155 = Build Array(w201) -> (w202:refnum<vi>[])
      n156 = call "Stopt VI.vi"("error in"=w204, "VI refnum"=w202) -> ("error out"=w203:errorcluster)  [unwired: 1 in]
    }
    frame #3 {
      # "Sense"
      n157 = vi-ref "Image Loop 1.vi"() -> (w205:refnum<vi>)
      n158 = vi-ref "Joypad Loop.vi"() -> (w206:refnum<vi>)
      n159 = vi-ref "Wiimote Loop.vi"() -> (w207:refnum<vi>)
      n160 = vi-ref "IMU Data Loop.vi"() -> (w208:refnum<vi>)
      n161 = vi-ref "VFH Visualization.vi"() -> (w212:refnum<vi>)
      n162 = vi-ref "About Robot.vi"() -> (w211:refnum<vi>)
      n163 = vi-ref "New GPS Data Loop.vi"() -> (w210:refnum<vi>)
      n164 = vi-ref "LIDAR Data Loop.vi"() -> (w209:refnum<vi>)
      n165 = Build Array(w205, w206, w207, w208, w212, w211, w210, w209) -> (w213:refnum<vi>[])
      n166 = call "Stopt VI.vi"("error in"=w215, "VI refnum"=w213) -> ("error out"=w214:errorcluster)  [unwired: 1 in]
    }
    frame #4 {
      # "Data  Log"
      n167 = vi-ref "Data Logging.vi"() -> (w218:refnum<vi>)
      n168 = vi-ref "Error UI.vi"() -> (w216:refnum<vi>)
      n169 = Build Array(w216, w218) -> (w219:refnum<vi>[])
      n170 = call "Stopt VI.vi"("error in"=w217, "VI refnum"=w219) -> ("error out"=w220:errorcluster)  [unwired: 1 in]
    }
    frame #5 {
      n171 = call <vilib>:"Simple Error Handler.vi"("error in (no error)"=w221) -> ()  [unwired: 4 in, 5 out]
    }
  }
